vi "geoAPI.vi"() -> (3 "Cluster 2":T1)   [LabVIEW 2018]
uses:
  <vilib>/Utility/error.llb/DialogType.ctl
  <vilib>/httpClient/LabVIEWHTTPClient.lvlib
  <vilib>/addons/_JKI.lib/Serialization/JSON/JKI JSON Serialization.lvlib
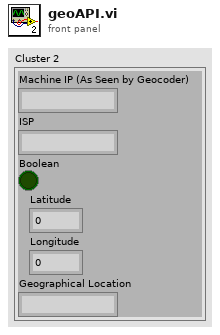
[diagram p1: front panel]
types:
  T1 = cluster{"Machine IP (As Seen by Geocoder)":string, "ISP":string, "Boolean":bool, "Latitude":dbl, "Longitude":dbl, "Geographical Location":string}
  T2 = cluster{"query":string, "isp":string, "status":string, "lat":dbl, "lon":dbl, "city":string, "regionName":string, "country":string, "zip":string}
  T3 = typedef "DialogType.ctl" = u16
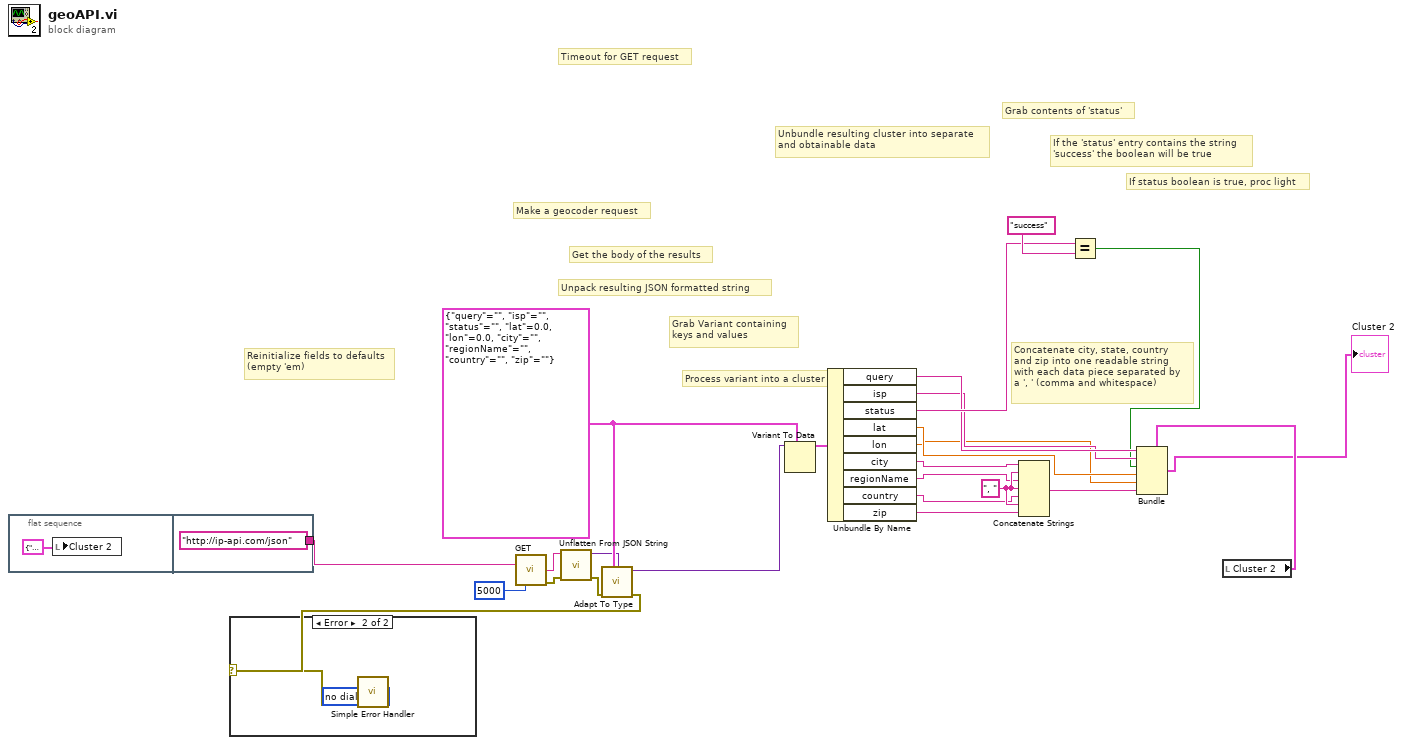
[diagram p0: block diagram]
diagram:
  w24 = ", "
  w20 = T2 {"query"="", "isp"="", "status"="", "lat"=0.0, "lon"=0.0, "city"="", "regionName"="", "country"="", "zip"=""}
  # "Reinitialize fields to defaults\n(empty 'em)"
  # "If status boolean is true, proc light"
  # "If the 'status' entry contains the string\n'success' the boolean will be true"
  # "Grab contents of 'status'"
  # "Concatenate city, state, country\nand zip into one readable string\nwith each data piece separated by\na ', ' (comma and whitespace)"
  # "Unbundle resulting cluster into separate\nand obtainable data"
  # "Process variant into a cluster"
  # "Grab Variant containing\nkeys and values"
  # "Unpack resulting JSON formatted string"
  # "Get the body of the results"
  # "Timeout for GET request"
  # "Make a geocoder request"
  n1 = flat-sequence {
    tunnel: ["http://ip-api.com/json"] -> w7
    frame #0 {
      n2 = local write "Cluster 2"(T1 {"Machine IP (As Seen by Geocoder)"="", "ISP"="", "Boolean"=FALSE, "Latitude"=0.0, "Longitude"=0.0, "Geographical Location"=""} ("Cluster 2")) -> ()
    }
    frame #1 {
    }
  }
  n3 = call <vilib>:"GET.vi"("url"=w7, "timeout (10000)"=5000) -> ("body"=w18:string, "error out"=w12:errorcluster)  [unwired: 10 in, 2 out]
  n4 = call <vilib>:"Unflatten From JSON String.vi"("error in (no error)"=w12, "JSON String"=w18) -> ("error out"=w11:errorcluster, "Variant"=w16:variant)  [unwired: 8 in]
  n5 = call <vilib>:"Adapt To Type.vi"("Type and Defaults"=w20, "error in (no error)"=w11, "Variant in"=w16) -> ("error out"=w10:errorcluster, "Variant out"=w17:variant)  [unwired: 7 in]
  n6 = case shown="Error" w10 {
    selector: w10 -> [_ w29]
    frame No Error {
    }
    frame Error {
      w28 = T3 0 items=["no dialog", "OK message", "continue or stop message", "OK message + warnings", "continue/stop + warnings"] ("type of dialog (OK msg:1)")
      n7 = call <vilib>:"Simple Error Handler.vi"("type of dialog (OK msg:1)"=w28, "error in (no error)"=w29) -> ()  [unwired: 3 in, 5 out]
    }
  }
  n8 = Variant To Data(type=w20, Variant=w17) -> (data=w19:T2)  [unwired: 1 in, 1 out]
  n9 = Unbundle By Name(w19) -> ("query"=w8:string, "isp"=w5:string, "status"=w13:string, "lat"=w3:dbl, "lon"=w2:dbl, "city"=w21:string, "regionName"=w22:string, "country"=w23:string, "zip"=w25:string)
  n10 = Concatenate Strings(w21, w24, w22, w24, w23, w24, w25) -> (w1:string)
  n11 = Equal?(x=w13, y="success") -> (x = y?=w4:bool)
  n12 = local read "Cluster 2"() -> (w9:T1)
  n13 = Bundle(cluster=w9, "Machine IP (As Seen by Geocoder)"=w8, "ISP"=w5, "Boolean"=w4, "Latitude"=w3, "Longitude"=w2, "Geographical Location"=w1) -> (→"Cluster 2":T1)
